vi "Fluke Multimeter.vi"(8 "error in (no error)":errorcluster, 11 "Fluke Multimeter in":refnum<class "Fluke Multimeter.lvclass">) -> (0 "error out":errorcluster, 3 "Fluke Multimeter out":refnum<class "Fluke Multimeter.lvclass">)   [LabVIEW 2009, in "Fluke Multimeter.lvclass"]
uses:
  Fluke Multimeter.lvclass
  Global/GPIB Numbers.vi
panel:
  out "Status":string
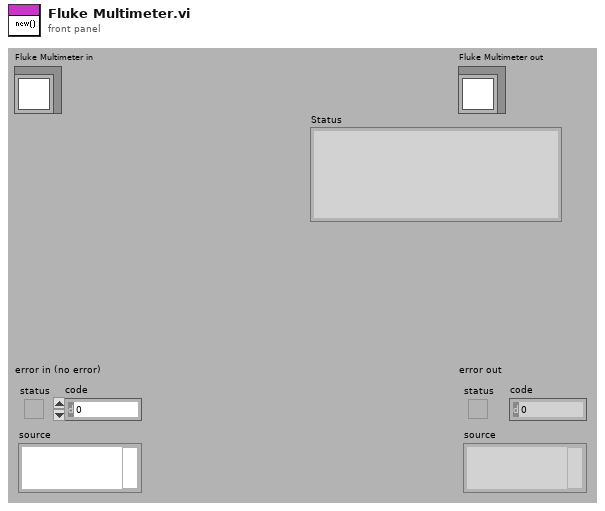
[diagram p1: front panel]
types:
  T1 = typedef "GPIB Type Def.ctl" = cluster{"Name":string, "bus":dbl, "GPIB":dbl, "GPIB as string":string, "byte":i32, "VISA Resource Name":refnum<visa-resource-name>}
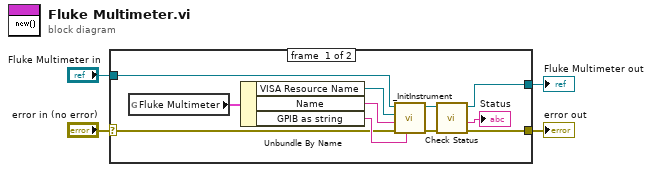
[diagram p0: block diagram]
diagram:
  n1 = case shown="No Error" "error in (no error)" {
    selector: "error in (no error)" -> [w7 w17]
    tunnel: [w6 w17] -> w3
    tunnel: [w12 w16] -> w1
    tunnel: "Fluke Multimeter in" -> [w13 w16]
    frame #0 {
      n2 = global read "GPIB Numbers.vi" "Fluke Multimeter"() -> (w15:T1)
      n3 = Unbundle By Name(w15) -> ("VISA Resource Name"=w11:refnum<visa-resource-name>, "Name"=w10:string, "GPIB as string"=w9:string)
      n4 = call-dynamic "_InitInstrument.vi"("GPIB as string"=w9, "error in (no error)"=w7, "Name"=w10, "VISA Resource Name"=w11, "Instrument in"=w13) -> ("error out"=w8:errorcluster, "Instrument out"=w14:refnum<class "Fluke Multimeter.lvclass">)  [unwired: 1 in, 4 out]
      n5 = call-dynamic "Check Status.vi"("error in (no error)"=w8, "Fluke Multimeter in"=w14) -> ("error out"=w6:errorcluster, "Status"=→"Status":string, "Fluke Multimeter out"=w12:refnum<class "Fluke Multimeter.lvclass">)  [unwired: 7 out]
    }
    frame #1 {
    }
  }
  "error out" <- w3
  "Fluke Multimeter out" <- w1
